vi "ComPortStructInit.vi"(10 "ComPort":refnum<visa-resource-name>) -> (5 "ComCluster out":T1)   [LabVIEW 2019]
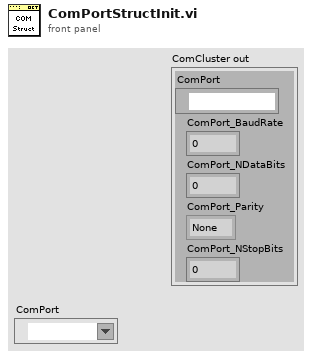
[diagram p1: front panel]
types:
  T1 = cluster{"ComPort":refnum<visa-resource-name>, "ComPort_BaudRate":u32, "ComPort_NDataBits":u16, "ComPort_Parity":enum16{"None", "Odd", "Even", "Mark", "Space"}, "ComPort_NStopBits":u16}
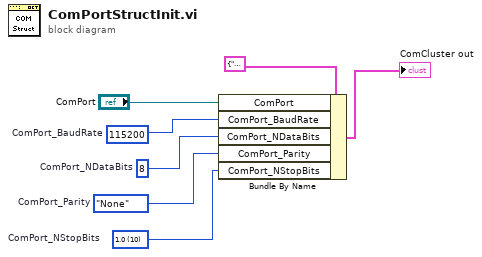
[diagram p0: block diagram]
diagram:
  w1 = u16 10 items=["1.0"=10, "1.5"=15, "2.0"=20]  # ComPort_NStopBits
  w3 = enum16{"None", "Odd", "Even", "Mark", "Space"}."None"  # ComPort_Parity
  w4 = u16 8  # ComPort_NDataBits
  w5 = u32 115200  # ComPort_BaudRate
  n1 = Bundle By Name(cluster=T1 {"ComPort"="", "ComPort_BaudRate"=0, "ComPort_NDataBits"=0, "ComPort_Parity"=enum."None", "ComPort_NStopBits"=0} ("ComCluster in in"), "ComPort"="ComPort", "ComPort_BaudRate"=w5, "ComPort_NDataBits"=w4, "ComPort_Parity"=w3, "ComPort_NStopBits"=w1) -> (→"ComCluster out":T1)
